vi "Sparse - Split Problem.vi"(8 "error in (no error)":errorcluster, 9 "Seed (-1)":i32=-1, 10 "Validation fraction":dbl=0.2 caption="Validation fraction (0.2)" format="%#_13g", 11 "svm_problem":T1) -> (0 "error out":errorcluster, 1 "Training indices":i32[](array[numeric]), 2 "Validation set":T1, 3 "Training set":T1, 5 "Validation indices":i32[](array[numeric]))   [LabVIEW 2015]
doc: "Splits the problem into a validation and training set, taking the amount of samples per class into account."
uses:
  LibSVM Sparse/Wrapper API/Controls/svm_problem.ctl
  LibSVM Sparse/Wrapper API/Controls/svm_node.ctl
  <vilib>/Analysis/1siggen.llb/Riffle Array (I32).vi
  <vilib>/Analysis/NI_AALBase.lvlib
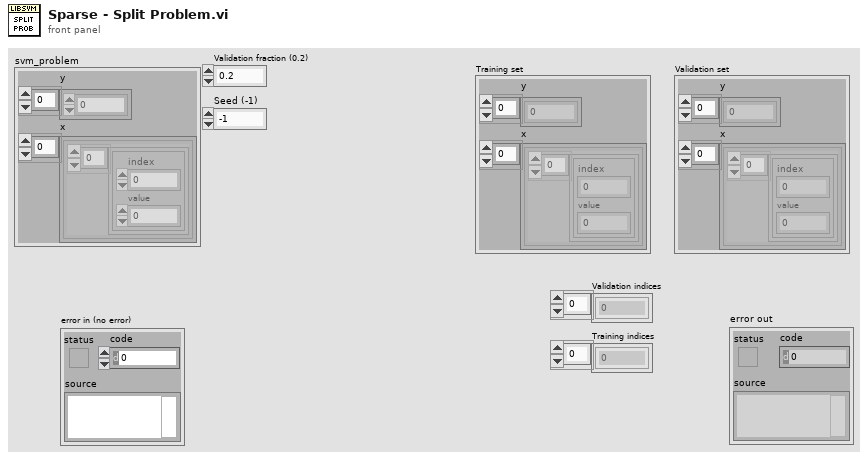
[diagram p1: front panel]
types:
  T1 = typedef "svm_problem.ctl" = cluster{"y":dbl[], "x":cluster{T2[]}[]}
  T2 = typedef "svm_node.ctl" = cluster{"index":i32, "value":dbl}
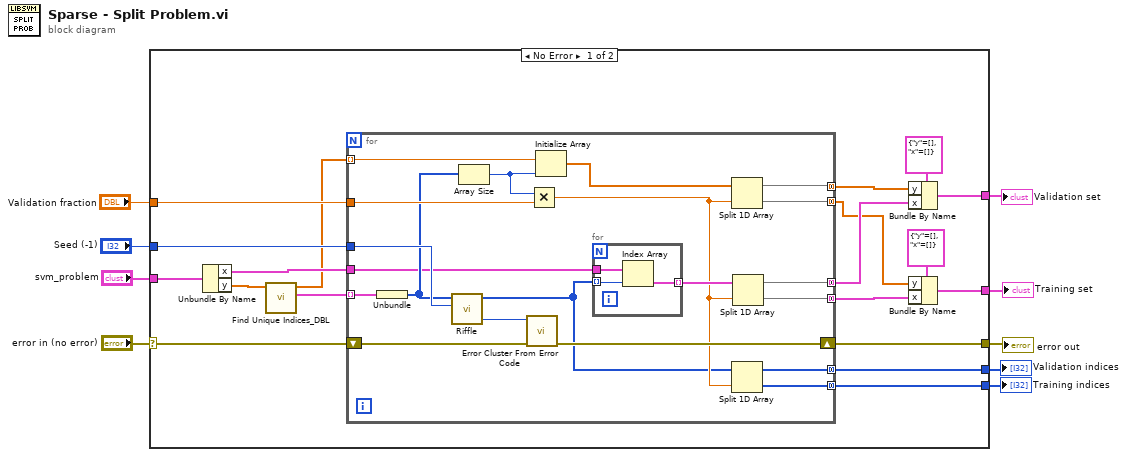
[diagram p0: block diagram]
diagram:
  n1 = case shown="No Error" "error in (no error)" {
    selector: "error in (no error)" -> [w24 w52]
    tunnel: [w14 w52] -> w9
    tunnel: "svm_problem" -> [w28 _]
    tunnel: "Seed (-1)" -> [w25 _]
    tunnel: "Validation fraction" -> [w22 _]
    tunnel: [w13 _] -> w4
    tunnel: [w12 _] -> w3
    tunnel: [w11 _] -> w2
    tunnel: [w10 _] -> w1
    frame No Error {
      n2 = Unbundle By Name(w28) -> ("x"=w23:cluster{T2[]}[], "y"=w27:dbl[])
      n3 = call "Find Unique Indices_DBL.vi"("Input Array"=w27) -> ("Unique indices"=w26:cluster{i32[]}[], "Unique values"=w21:dbl[])  [unwired: 9 in]
      n4 = for {
        tunnel: w26 -> [w48] mode=indexing
        tunnel: w25 -> [w47]
        shift-right: [w46] -> w14
        shift-left: w24 -> [w45]
        tunnel: w23 -> [w41]
        tunnel: w22 -> [w43]
        tunnel: [w39] -> w17 mode=concatenating
        tunnel: [w38] -> w15 mode=concatenating
        tunnel: w21 -> [w37] mode=indexing
        tunnel: [w34] -> w18 mode=concatenating
        tunnel: [w33] -> w16 mode=concatenating
        tunnel: [w31] -> w11 mode=concatenating
        tunnel: [w30] -> w10 mode=concatenating
        n5 = Unbundle(w48) -> (w42:i32[])
        n6 = call-poly <vilib>:"Riffle.vi"("seed"=w47, "X"=w42) -> ("error"=w44:i32, "Riffled {X}"=w29:i32[])  [unwired: 7 in, 1 out]
        n7 = Array Size(array=w42) -> (size(s)=w36:i32)
        n8 = call <vilib>:"Error Cluster From Error Code.vi"("error in (no error)"=w45, "error code (0)"=w44) -> ("error out"=w46:errorcluster)  [unwired: 7 in]
        n9 = Multiply(x=w36, y=w43) -> (x*y=w32:dbl)
        n10 = Initialize Array(w37, w36) -> (w35:dbl[])
        n11 = for {
          tunnel: w29 -> [w50] mode=indexing
          tunnel: w41 -> [w51]
          tunnel: [w49] -> w40 mode=indexing
          n12 = Index Array(array=w51, index=w50) -> (element=w49:cluster{T2[]})
        }
        n13 = Split 1D Array(array=w35, index=w32) -> (first subarray=w34:dbl[], second subarray=w33:dbl[])
        n14 = Split 1D Array(array=w29, index=w32) -> (first subarray=w31:i32[], second subarray=w30:i32[])
        n15 = Split 1D Array(array=w40, index=w32) -> (first subarray=w39:cluster{T2[]}[], second subarray=w38:cluster{T2[]}[])
      }
      n16 = Bundle By Name(cluster=T1 {"y"=[], "x"=[]} ("svm_problem"), "y"=w18, "x"=w17) -> (w12:T1)
      n17 = Bundle By Name(cluster=T1 {"y"=[], "x"=[]} ("svm_problem"), "y"=w16, "x"=w15) -> (w13:T1)
    }
    frame Error {
    }
  }
  "error out" <- w9
  "Training set" <- w4
  "Validation set" <- w3
  "Validation indices" <- w2
  "Training indices" <- w1
